vi "AlliGator Add Test Result.vi"(8 "error in (no error)":errorcluster) -> (0 "error out":errorcluster)   [LabVIEW 2021, in "AlliGator Test Suite.lvlib"]
uses:
  AlliGator Test Data.ctl
  AlliGator Test Suite.lvlib
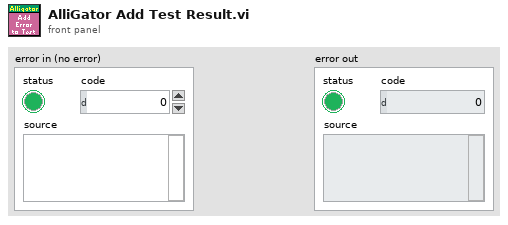
[diagram p1: front panel]
types:
  T1 = enum16{"Store Test Name", "Store Test Result", "Read Test Result"}
  T2 = typedef "AlliGator Test Suite.lvlib/AlliGator Test Data.ctl" = cluster{"Test String":string, "error":errorcluster, "Status":bool}
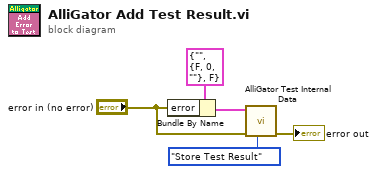
[diagram p0: block diagram]
diagram:
  n1 = Bundle By Name(cluster=T2 {"Test String"="", "error"={"status"=FALSE, "code"=0, "source"=""}, "Status"=FALSE} ("AlliGator Test Data"), "error"="error in (no error)") -> (w3:T2)
  n2 = call "AlliGator Test Internal Data.vi"("Test State"=T1."Store Test Result", "Error In"="error in (no error)", "AlliGator Test Data"=w3) -> ("Error Out"=→"error out":errorcluster)  [unwired: 7 in, 1 out]
